vi "MGCC_FntStaMach_Initialization.vi"   [LabVIEW 2016]
doc: "This VI is used to initize the events and flags in the FSM. In the future, it may be used to initize the variables in other function VIs."
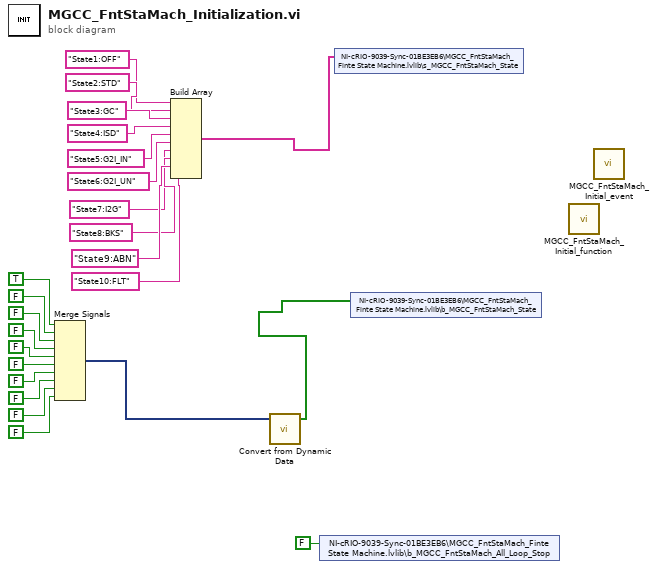
[diagram p0: block diagram]
diagram:
  n1 = Merge Signals(TRUE ("State3"), FALSE ("State3"), FALSE ("State3"), FALSE ("State3"), FALSE ("State3"), FALSE ("State3"), FALSE ("State3"), FALSE ("State3"), FALSE ("State3"), FALSE ("State3")) -> (w14:dynamicdata)
  n2 = Build Array("State1:OFF", "State2:STD", "State3:GC", "State4:ISD", "State5:G2I_IN", "State6:G2I_UN", "State7:I2G", "State8:BKS", "State9:ABN", "State10:FLT") -> (w3:string[])
  n3 = call "Convert from Dynamic Data"("Dynamic Data Type"=w14) -> ("Array"=w2:bool[])  [unwired: 3 in]
  n4 = shared-variable "NI-cRIO-9039-Sync-01BE3EB6\\MGCC_FntStaMach_Finte State Machine.lvlib\\b_MGCC_FntStaMach_All_Loop_Stop"(FALSE ("ALL loop stop")) -> ()  [unwired: 1 in, 1 out]
  n5 = shared-variable "NI-cRIO-9039-Sync-01BE3EB6\\MGCC_FntStaMach_Finte State Machine.lvlib\\s_MGCC_FntStaMach_State"(w3) -> ()  [unwired: 1 in, 1 out]
  n6 = shared-variable "NI-cRIO-9039-Sync-01BE3EB6\\MGCC_FntStaMach_Finte State Machine.lvlib\\b_MGCC_FntStaMach_State"(w2) -> ()  [unwired: 1 in, 1 out]
  n7 = call "MGCC_FntStaMach_Initial_function.vi"() -> ()  [unwired: 12 in]
  n8 = call "MGCC_FntStaMach_Initial_event.vi"() -> ()  [unwired: 12 in]
